vi "C400 Example.vi"() -> ()   [LabVIEW 2017]
panel:
  in  "phase":dbl format="%.2p"
  in  "frequency":dbl=1.0 format="%0.2p"
  in  "amplitude":dbl=10.0 format="%0.2p"
  in  "signal type":T1(ring)
  in  "offset":dbl format="%0.2p"
  in  "Stop Waveform":bool
  in  "Start Waveform":bool
  in  "Run Chart":bool
  out "Sensor Reading Waveform Chart":dbl(graph)=-15.449458025852254
  out "Ch1 Position Units":string
  out "Ch1Range":i32
  in  "Read Sensor":bool
  out "Ch1 Sensor Value":dbl format="%.3f"
  out "Serial Number Array":string[](array[string])
  out "FT_Status":u64(ring) items=["FT_OK", "FT_INVALID_HANDLE", "FT_DEVICE_NOT_FOUND", "FT_DEVICE_NOT_OPENED", "FT_IO_ERROR", "FT_INSUFFICIENT_RESOURCES", "FT_INVALID_PARAMETER", "FT_INVALID_BAUD_RATE", "FT_DEVICE_NOT_OPENED_FOR_ERASE", "FT_DEVICE_NOT_OPENED_FOR_WRITE", "FT_FAILED_TO_WRITE_DEVICE", "FT_EEPROM_READ_FAILED", "FT_EEPROM_WRITE_FAILED", "FT_EEPROM_ERASE_FAILED", "FT_EEPROM_NOT_PRESENT", "FT_EEPROM_NOT_PROGRAMMED", "FT_INVALID_ARGS", "FT_NOT_SUPPORTED", "FT_OTHER_ERROR"]
  in  "Ch1 Position Cmd":dbl format="%.3f"
  in  "Connect":bool
  in  "Stop Button":bool
  in  "Listbox":i32(listbox)=-1
  in  "Handle":u64
  # "Waveform Controls"
  # "FT_Status displays the error type if an\nFTDI USB function did not execute properly."
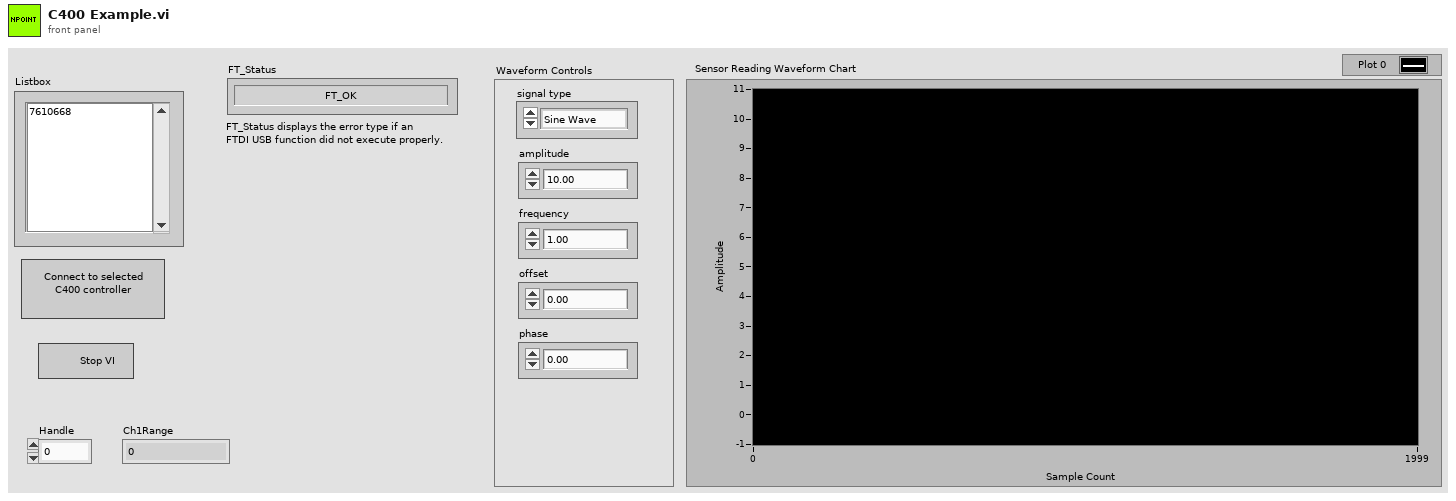
[diagram p1: front panel]
types:
  T1 = enum16{"Sine Wave", "Triangle Wave", "Square Wave", "Sawtooth Wave"}
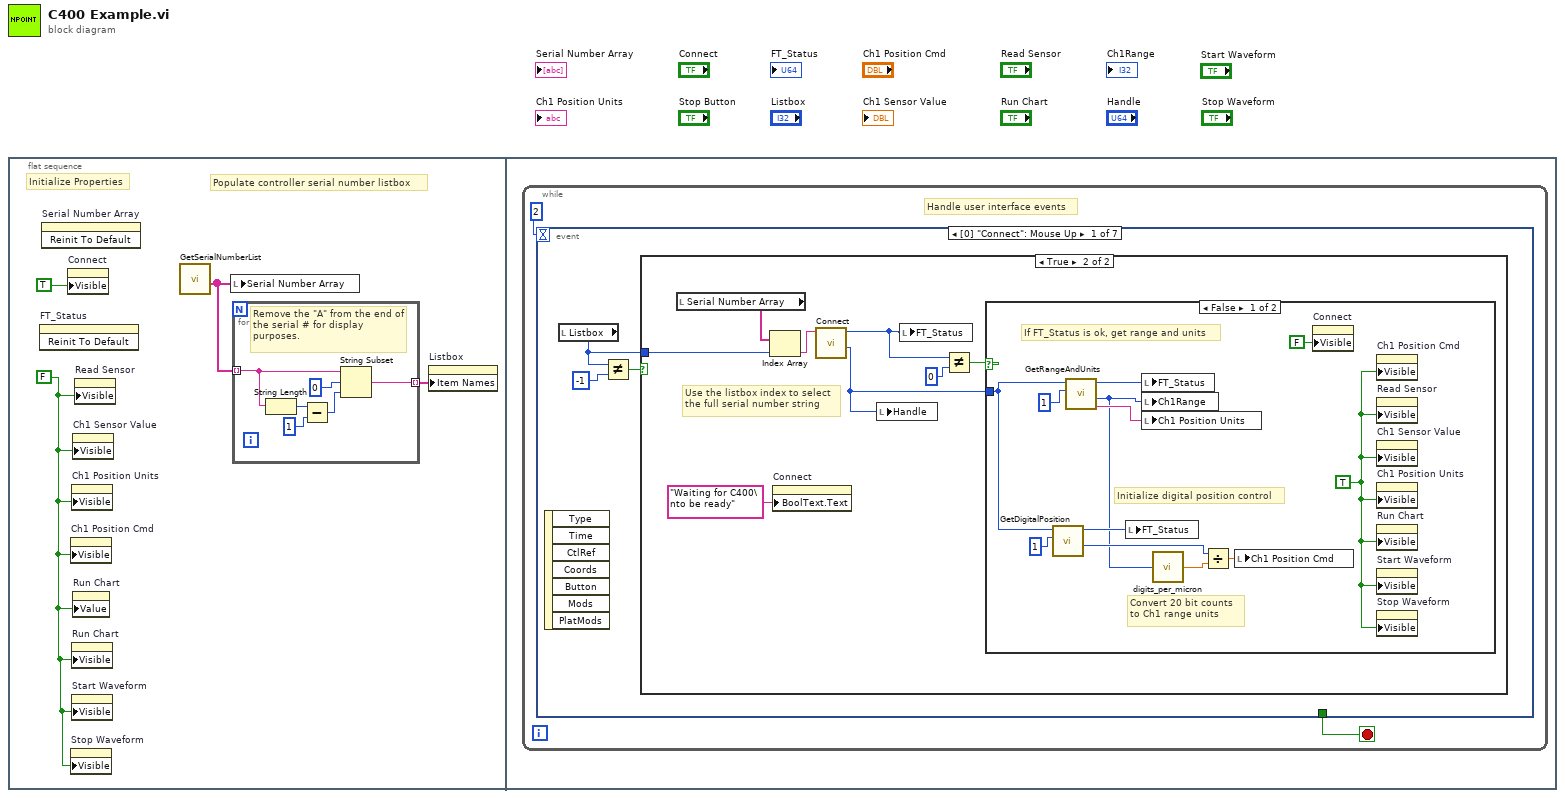
[diagram p0: block diagram]
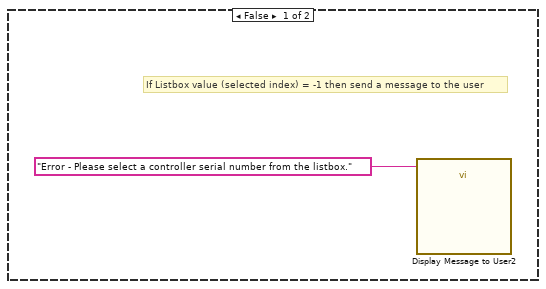
[diagram p2: hidden frame]
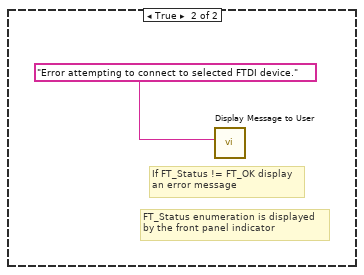
[diagram p3: hidden frame]
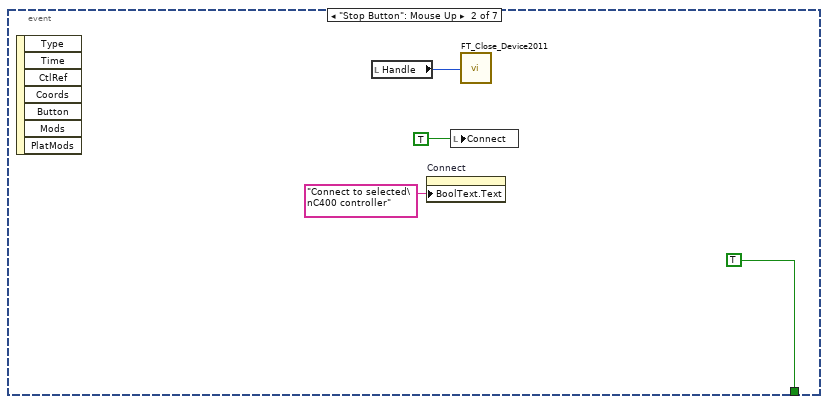
[diagram p4: hidden frame]
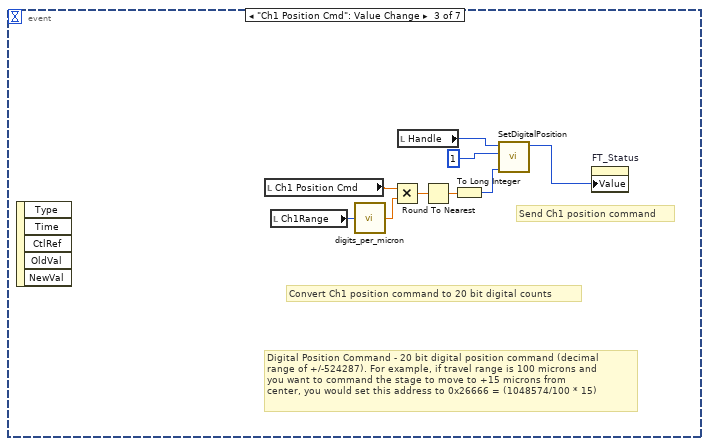
[diagram p5: hidden frame]
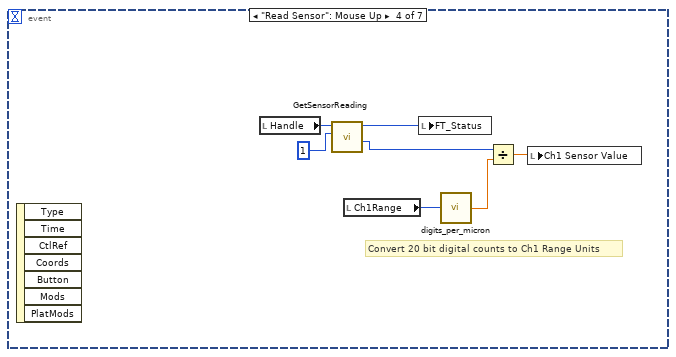
[diagram p6: hidden frame]
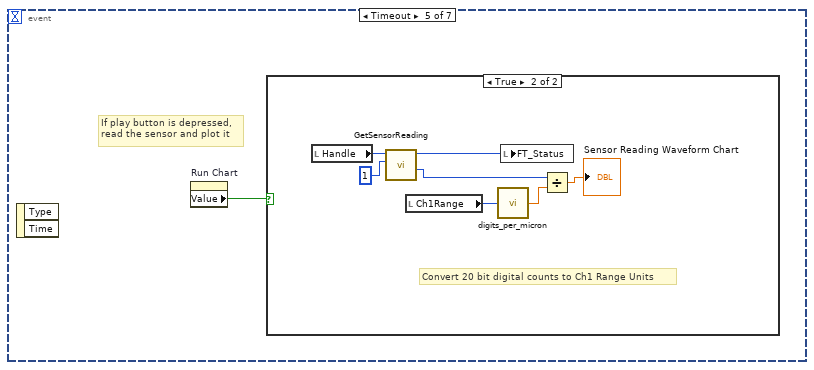
[diagram p7: hidden frame]
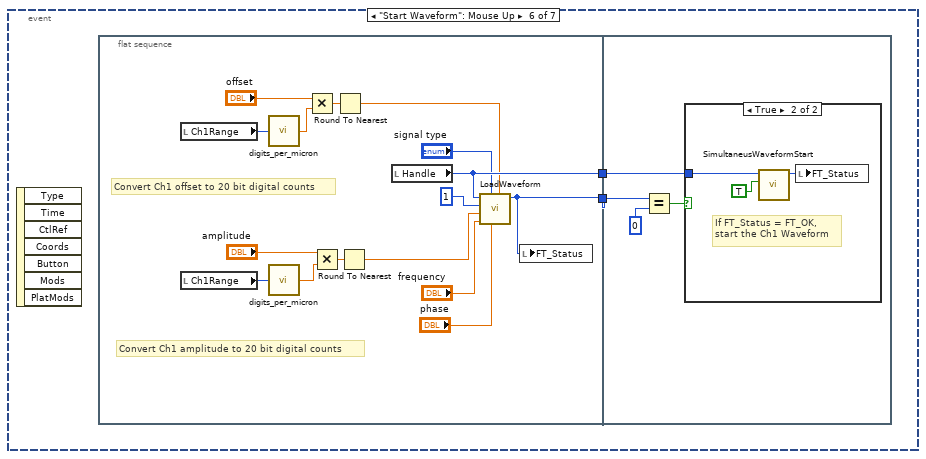
[diagram p9: hidden frame]
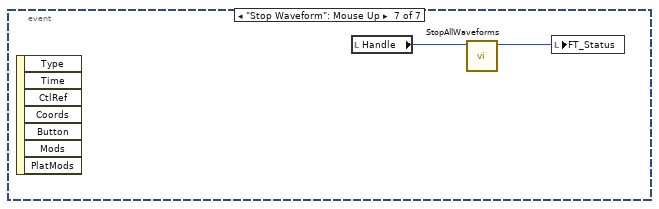
[diagram p11: hidden frame]
diagram:
  n1 = flat-sequence {
    frame #0 {
      w1 = FALSE ("Visible")
      # "Initialize Properties"
      # "Populate controller serial number listbox"
      n2 = invoke on="FT_Status" class="Ring (strict)" method="Reinit To Default"() -> ()  [unwired: 3 in, 3 out]
      n3 = invoke on="Serial Number Array" class="Arr (strict)" method="Reinit To Default"() -> ()  [unwired: 3 in, 3 out]
      n4 = property on="Connect" class="Bool (strict)"("Visible"=TRUE) -> ()  [unwired: 2 in, 2 out]
      n5 = property on="Ch1 Position Cmd" class="DigNum (strict)"("Visible"=w1) -> ()  [unwired: 2 in, 2 out]
      n6 = property on="Stop Waveform" class="Bool (strict)"("Visible"=w1) -> ()  [unwired: 2 in, 2 out]
      n7 = property on="Ch1 Position Units" class="Str"("Visible"=w1) -> ()  [unwired: 2 in, 2 out]
      n8 = property on="Run Chart" class="Bool (strict)"("Visible"=w1) -> ()  [unwired: 2 in, 2 out]
      n9 = property on="Start Waveform" class="Bool (strict)"("Visible"=w1) -> ()  [unwired: 2 in, 2 out]
      n10 = property on="Ch1 Sensor Value" class="DigNum (strict)"("Visible"=w1) -> ()  [unwired: 2 in, 2 out]
      n11 = property on="Run Chart" class="Bool (strict)"("Value"=w1) -> ()  [unwired: 2 in, 2 out]
      n12 = property on="Read Sensor" class="Bool (strict)"("Visible"=w1) -> ()  [unwired: 2 in, 2 out]
      n13 = call "GetSerialNumberList.vi"() -> ("C400 Serial Number Array"=w3:string[])  [unwired: 11 in]
      n14 = local write "Serial Number Array"(w3) -> ()
      n15 = for {
        tunnel: [w6] -> w4 mode=indexing
        tunnel: w3 -> [w5] mode=indexing
        # "Remove the \"A\" from the end of the serial # for display purposes."
        n16 = String Length(string=w5) -> (length=w9:i32)
        n17 = Subtract(x=w9, y=1) -> (x-y=w7:i32)
        n18 = String Subset(string=w5, offset (0)=0, length (rest)=w7) -> (substring=w6:string)
      }
      n19 = property on="Listbox" class="LstBox (strict)"("Item Names"=w4) -> ()  [unwired: 2 in, 2 out]
    }
    frame #1 {
      n20 = while {
        stop <- w12 stop-if-true
        # "Handle user interface events"
        n21 = event shown="[0] \"Connect\": Mouse Up" {
          selector: _ -> [_ _ _ _ _ _ _]
          dyn-events: _ -> [_ _ _ _ _ _ _]
          timeout: 2 -> [_ _ _ _ _ _ _]
          tunnel: [_ TRUE _ _ _ _ _] -> w12
          event "Connect": Mouse Up {
            n22 = event-data() -> ()  [unwired: 1 in, 7 out]
            n23 = local read "Listbox"() -> (w13:i32)
            n24 = Not Equal?(x=w13, y=-1) -> (x != y?=w15:bool)
            n25 = case shown="True" w15 {
              tunnel: w13 -> [_ w24]
              frame False {
                # "If Listbox value (selected index) = -1 then send a message to the user"
                n26 = call "Display Message to User2"("Message"="Error - Please select a controller serial number from the listbox.") -> ()  [unwired: 9 in, 2 out]
              }
              frame True {
                # "Use the listbox index to select\nthe full serial number string"
                n27 = local read "Serial Number Array"() -> (w19:string[])
                n28 = Index Array(array=w19, index=w24) -> (element=w20:string)
                n29 = property on="Connect" class="Bool (strict)"("BoolText.Text"="Waiting for C400\nto be ready" ("Boolean Text.Text")) -> ()  [unwired: 2 in, 2 out]
                n30 = call "Connect.vi"("Device Serial Number"=w20) -> ("Handle"=w23:u64, "FT_Status"=w18:u64)  [unwired: 9 in]
                n31 = local write "Handle"(w23) -> ()
                n32 = local write "FT_Status"(w18) -> ()
                n33 = Not Equal?(x=w18, y=u64 0) -> (x != y?=w21:bool)
                n34 = case shown="False" w21 {
                  tunnel: w23 -> [w30 _]
                  frame False {
                    w27 = TRUE ("Visible")
                    # "Convert 20 bit counts\nto Ch1 range units"
                    # "Initialize digital position control"
                    # "If FT_Status is ok, get range and units"
                    n35 = call "GetDigitalPosition.vi"("Handle"=w30, "Controller Channel"=i64 1) -> ("FT_Status"=w28:u64, "Position"=w34:i64)  [unwired: 7 in]
                    n36 = call "GetRangeAndUnits.vi"("Handle"=w30, "Controller Channel"=i64 1) -> ("FT_Status"=w32:u64, "Range"=w25:i32, "Range Units"=w31:string)  [unwired: 6 in]
                    n37 = local write "FT_Status"(w28) -> ()
                    n38 = local write "FT_Status"(w32) -> ()
                    n39 = local write "Ch1Range"(w25) -> ()
                    n40 = local write "Ch1 Position Units"(w31) -> ()
                    n41 = call "digits_per_micron.vi"("Ch1Range"=w25) -> ("digital_per_micron"=w26:dbl)
                    n42 = Divide(x=w34, y=w26) -> (x/y=w29:dbl)
                    n43 = local write "Ch1 Position Cmd"(w29) -> ()
                    n44 = property on="Connect" class="Bool (strict)"("Visible"=FALSE) -> ()  [unwired: 2 in, 2 out]
                    n45 = property on="Ch1 Position Cmd" class="DigNum (strict)"("Visible"=w27) -> ()  [unwired: 2 in, 2 out]
                    n46 = property on="Read Sensor" class="Bool (strict)"("Visible"=w27) -> ()  [unwired: 2 in, 2 out]
                    n47 = property on="Ch1 Sensor Value" class="DigNum (strict)"("Visible"=w27) -> ()  [unwired: 2 in, 2 out]
                    n48 = property on="Ch1 Position Units" class="Str"("Visible"=w27) -> ()  [unwired: 2 in, 2 out]
                    n49 = property on="Run Chart" class="Bool (strict)"("Visible"=w27) -> ()  [unwired: 2 in, 2 out]
                    n50 = property on="Start Waveform" class="Bool (strict)"("Visible"=w27) -> ()  [unwired: 2 in, 2 out]
                    n51 = property on="Stop Waveform" class="Bool (strict)"("Visible"=w27) -> ()  [unwired: 2 in, 2 out]
                  }
                  frame True {
                    # "FT_Status enumeration is displayed\nby the front panel indicator"
                    # "If FT_Status != FT_OK display\nan error message"
                    n52 = call "Display Message to User"("Message"="Error attempting to connect to selected FTDI device.") -> ()  [unwired: 9 in, 2 out]
                  }
                }
              }
            }
          }
          event "Stop Button": Mouse Up {
            n53 = event-data() -> ()  [unwired: 1 in, 7 out]
            n54 = local read "Handle"() -> (w39:u64)
            n55 = property on="Connect" class="Bool (strict)"("BoolText.Text"="Connect to selected\nC400 controller" ("Boolean Text.Text")) -> ()  [unwired: 2 in, 2 out]
            n56 = local write "Connect"(TRUE ("Visible")) -> ()
            n57 = call "FT_Close_Device2011.vi"("Handle"=w39) -> ()  [unwired: 1 out]
          }
          event "Ch1 Position Cmd": Value Change {
            # "Digital Position Command - 20 bit digital position command (decimal\nrange of +/-524287). For example, if travel range is 100 microns and\nyou want to command the stage to move to +15 microns from\ncenter, you would set this address to 0x26666 = (1048574/100 * 15)"
            # "Send Ch1 position command"
            # "Convert Ch1 position command to 20 bit digital counts"
            n58 = event-data() -> ()  [unwired: 1 in, 5 out]
            n59 = local read "Ch1 Position Cmd"() -> (w44:dbl)
            n60 = local read "Ch1Range"() -> (w43:i32)
            n61 = call "digits_per_micron.vi"("Ch1Range"=w43) -> ("digital_per_micron"=w42:dbl)
            n62 = Multiply(x=w44, y=w42) -> (x*y=w48:dbl)
            n63 = local read "Handle"() -> (w45:u64)
            n64 = Round To Nearest(number=w48) -> (nearest integer value=w47:dbl)
            n65 = To Long Integer(number=w47) -> (32bit integer=w46:i32)
            n66 = call "SetDigitalPosition.vi"("Position"=w46, "Controller Channel"=i64 1, "Handle"=w45) -> ("FT_Status"=w49:u64)  [unwired: 8 in]
            n67 = property on="FT_Status" class="Ring (strict)"("Value"=w49) -> ()  [unwired: 2 in, 2 out]
          }
          event "Read Sensor": Mouse Up {
            # "Convert 20 bit digital counts to Ch1 Range Units"
            n68 = event-data() -> ()  [unwired: 1 in, 7 out]
            n69 = local read "Handle"() -> (w54:u64)
            n70 = call "GetSensorReading.vi"("Handle"=w54, "Controller Channel"=i64 1) -> ("FT_Status"=w55:u64, "Sensor Reading"=w56:i64)  [unwired: 7 in]
            n71 = local read "Ch1Range"() -> (w51:i32)
            n72 = local write "FT_Status"(w55) -> ()
            n73 = call "digits_per_micron.vi"("Ch1Range"=w51) -> ("digital_per_micron"=w52:dbl)
            n74 = Divide(x=w56, y=w52) -> (x/y=w53:dbl)
            n75 = local write "Ch1 Sensor Value"(w53) -> ()
          }
          event Timeout {
            # "If play button is depressed,\nread the sensor and plot it"
            n76 = event-data() -> ()  [unwired: 1 in, 2 out]
            n77 = property on="Run Chart" class="Bool (strict)"() -> ("Value"=w58:bool)  [unwired: 2 in, 2 out]
            n78 = case shown="True" w58 {
              frame False {
              }
              frame True {
                # "Convert 20 bit digital counts to Ch1 Range Units"
                n79 = local read "Handle"() -> (w62:u64)
                n80 = call "GetSensorReading.vi"("Handle"=w62, "Controller Channel"=i64 1) -> ("FT_Status"=w61:u64, "Sensor Reading"=w64:i64)  [unwired: 7 in]
                n81 = local read "Ch1Range"() -> (w60:i32)
                n82 = call "digits_per_micron.vi"("Ch1Range"=w60) -> ("digital_per_micron"=w59:dbl)
                n83 = local write "FT_Status"(w61) -> ()
                n84 = Divide(x=w64, y=w59) -> (x/y=→"Sensor Reading Waveform Chart":dbl)
              }
            }
          }
          event "Start Waveform": Mouse Up {
            n85 = event-data() -> ()  [unwired: 1 in, 7 out]
            n86 = flat-sequence {
              tunnel: [w72] -> w67
              tunnel: [w83] -> w66
              tunnel: w67 -> [w87]
              tunnel: w66 -> [w84]
              frame #0 {
                # "Convert Ch1 offset to 20 bit digital counts"
                # "Convert Ch1 amplitude to 20 bit digital counts"
                n87 = local read "Ch1Range"() -> (w69:i32)
                n88 = local read "Ch1Range"() -> (w71:i32)
                n89 = call "digits_per_micron.vi"("Ch1Range"=w69) -> ("digital_per_micron"=w68:dbl)
                n90 = call "digits_per_micron.vi"("Ch1Range"=w71) -> ("digital_per_micron"=w70:dbl)
                n91 = Multiply(x="offset", y=w68) -> (x*y=w75:dbl)
                n92 = Multiply(x="amplitude", y=w70) -> (x*y=w78:dbl)
                n93 = Round To Nearest(number=w75) -> (nearest integer value=w73:dbl)
                n94 = Round To Nearest(number=w78) -> (nearest integer value=w76:dbl)
                n95 = local read "Handle"() -> (w83:u64)
                n96 = call "LoadWaveform.vi"("offset"=w73, "phase"="phase", "signal type"="signal type", "frequency"="frequency", "amplitude"=w76, "Channel"=i64 1 ("Controller Channel"), "Handle"=w83) -> ("FT_Status"=w72:u64)  [unwired: 4 in]
                n97 = local write "FT_Status"(w72) -> ()
              }
              frame #1 {
                n98 = Equal?(x=w87, y=u32 0) -> (x = y?=w85:bool)
                n99 = case shown="True" w85 {
                  tunnel: w84 -> [_ w89]
                  frame False {
                  }
                  frame True {
                    # "If FT_Status = FT_OK,\nstart the Ch1 Waveform"
                    n100 = call "SimultaneusWaveformStart.vi"("Ch1Start"=TRUE, "Handle"=w89) -> ("FT_Status"=w88:u64)  [unwired: 9 in]
                    n101 = local write "FT_Status"(w88) -> ()
                  }
                }
              }
            }
          }
          event "Stop Waveform": Mouse Up {
            n102 = event-data() -> ()  [unwired: 1 in, 7 out]
            n103 = local read "Handle"() -> (w92:u64)
            n104 = call "StopAllWaveforms.vi"("Handle"=w92) -> ("FT_Status"=w91:u64)  [unwired: 10 in]
            n105 = local write "FT_Status"(w91) -> ()
          }
        }
      }
    }
  }
